vi "Launcher.vi"() -> ()   [LabVIEW 2014]
uses:
  Project/Framework/ActorMeter/ActorMeter.lvclass
  Project/Framework/ActorMeter/ActorMeter.lvclass/ActorMeter.ctl
  <vilib>/ActorFramework/Actor/Actor.lvclass
panel:
  in  "Experiment type":string(combo)="WS_Real1D"
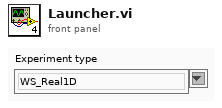
[diagram p1: front panel]
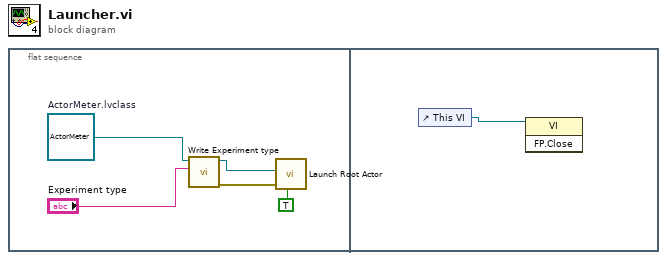
[diagram p0: block diagram]
diagram:
  n1 = flat-sequence {
    frame #0 {
      w1 = refnum<class "ActorMeter.lvclass"> refnum  # ActorMeter.lvclass
      n2 = call "Write Experiment type.vi"("Experiment type"="Experiment type", "ActorMeter in"=w1) -> ("error out"=w3:errorcluster, "ActorMeter out"=w2:refnum<class "ActorMeter.lvclass">)  [unwired: 8 in]
      n3 = call <vilib>:"Launch Root Actor.vi"("Open Actor Core front panel? (F)"=TRUE, "error in (no error)"=w3, "Actor"=w2) -> ()  [unwired: 7 in, 2 out]
    }
    frame #1 {
      n4 = control-ref of="This VI"() -> (w6:refnum<vi>)
      n5 = invoke class="VI" method="FP.Close"(reference=w6) -> ()  [unwired: 2 in, 3 out]
    }
  }
